vi "CtrlTrain_Analog_Rate.vi"(6 "Scale":dbl=1.0, 11 "Input":dbl) -> (3 "Output":dbl)   [LabVIEW 2019, in "CtrlTrainingLibary_Protected.lvlib"]
doc: "This VI rate limits the input. This VI remembers the last output. If there are multiple VI that set the same output, use the RateLimit2 VI. This one has an input connection to send the last output value."
uses:
  CtrlTrainingLibary_Protected.lvlib
  <vilib>/Rock Robotics/WPI/ThirdParty/JAS_Junk/TrajLib/Trajectory_Library.lvlib
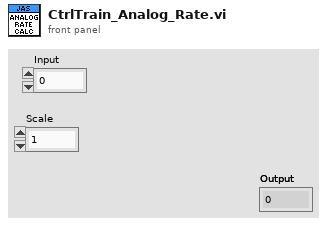
[diagram p1: front panel]
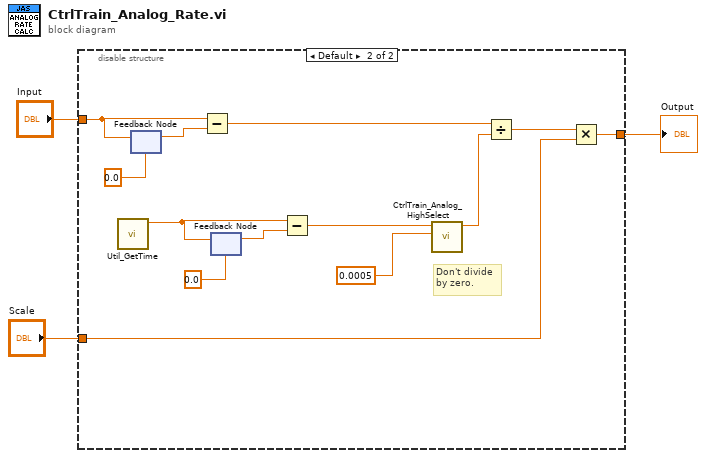
[diagram p0: block diagram]
diagram:
  n1 = disable-structure shown="Default" {
    disable-tunnel: "Input" -> [_ w15]
    disable-tunnel: "Scale" -> [_ w9]
    disable-tunnel: [_ w8] -> w1
    frame condition #0 {
    }
    frame condition #1 (active) {
      # "Don't divide\nby zero."
      n2 = call <vilib>:"Util_GetTime.vi"() -> ("FPGA_Time_Seconds"=w4:dbl)  [unwired: 10 in, 1 out]
      n3 = feedback #1(0.0 ("Input")) -> (w14:dbl)
      n4 = feedback-in #1(w15) -> ()
      n5 = Subtract(x=w15, y=w14) -> (x-y=w11:dbl)
      n6 = feedback #2(0.0 ("Input")) -> (w12:dbl)
      n7 = feedback-in #2(w4) -> ()
      n8 = Subtract(x=w4, y=w12) -> (x-y=w7:dbl)
      n9 = call "CtrlTrain_Analog_HighSelect.vi"("Input_2"=0.0005, "Input_1"=w7) -> ("Output"=w5:dbl)  [unwired: 9 in]
      n10 = Divide(x=w11, y=w5) -> (x/y=w10:dbl)
      n11 = Multiply(x=w10, y=w9) -> (x*y=w8:dbl)
    }
  }
  "Output" <- w1
